vi "Contador_2pi.vi"() -> ()   [LabVIEW 2016]
panel:
  out "Numeric Control":dbl
  in  "Stop Button":bool
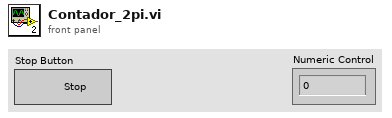
[diagram p1: front panel]
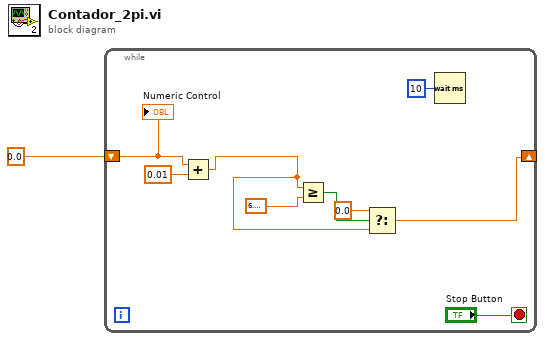
[diagram p0: block diagram]
diagram:
  n1 = while {
    shift-right: [w2] -> _
    shift-left: 0.0 -> [w10]
    stop <- "Stop Button" stop-if-true
    n2 = Add(x=w10, y=0.01) -> (x+y=w3:dbl)
    n3 = Greater Or Equal?(x=w3, y=6.283185307179586) -> (x >= y?=w5:bool)
    n4 = Select(t=0.0, s=w5, f=w3) -> (s? t:f=w2:dbl)
    n5 = Wait (ms)(milliseconds to wait=u32 10) -> ()  [unwired: 1 out]
    "Numeric Control" <- w10
  }
